vi "Derivative PCA Cycles (SubVI).vi"(8 "Derivative filter on?":bool=TRUE, 9 "Derivative LPF cutoff (Hz)":dbl=15.0, 10 "dt":dbl=50.0, 11 "Waveform (samples) in":dbl[](array[numeric])) -> (0 "AIx Related":T1={"Type (4th D ZC)"=enum."Type B", "AIx (%) (4th D ZC) "=9.808766983260572, "AP (mmHg)  (4th DZC)"=3.579441860465124}, 1 "Waveform Graph":dynamicdata(graph), 3 "Fid. Points (SDW)":T2)   [LabVIEW 2017]
uses:
  <vilib>/Analysis/NI_AAL_SigProc.lvlib
panel:
  out "SDW ZC2":dbl
  out "FoDW (Peaks)":dbl[](array[numeric])
  out "FDW (Peaks)":dbl[](array[numeric])=[27.628093409204006, 83.82448575360515, 357.5002701435206, 373.0498792154545]
  out "SDW (Peaks)":dbl[](array[numeric])
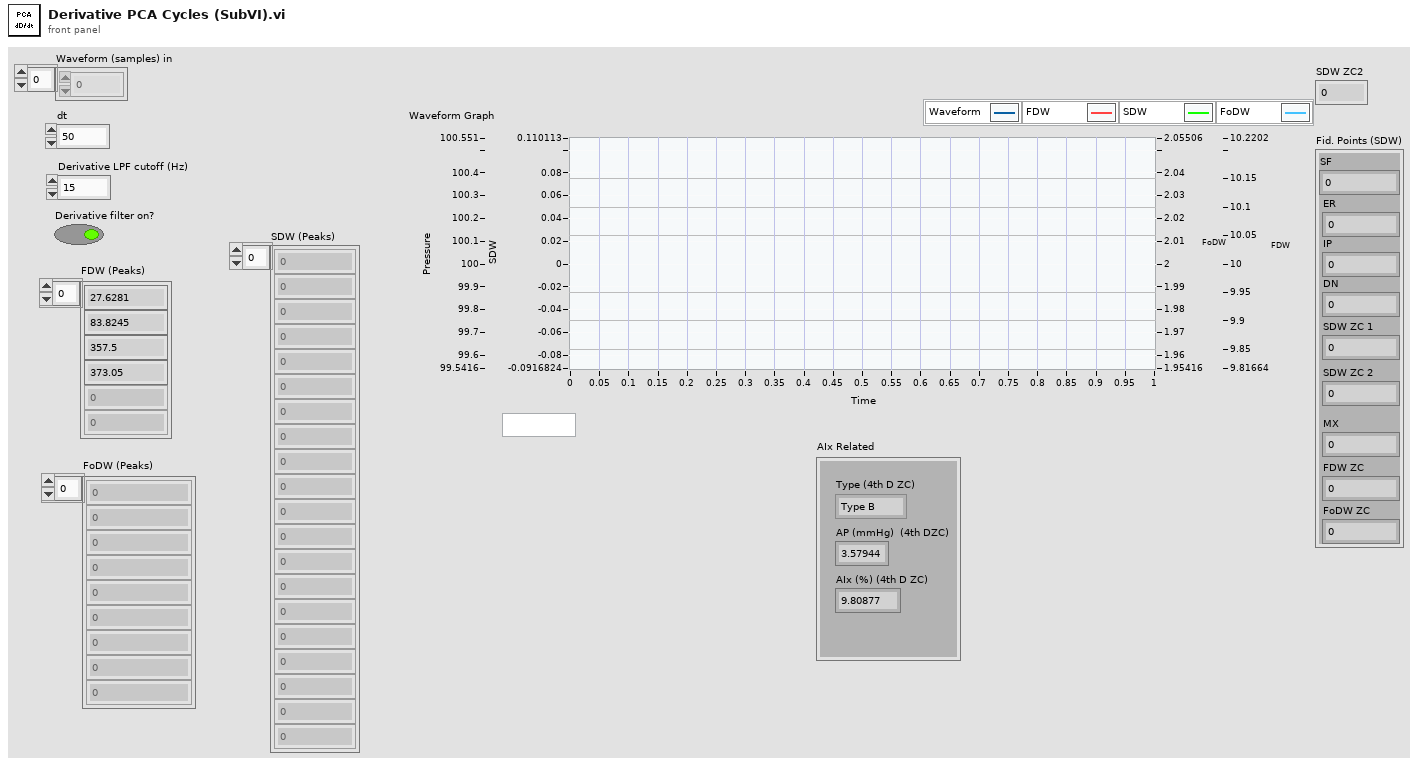
[diagram p1: front panel]
types:
  T1 = cluster{"Type (4th D ZC)":enum16{"Type A", "Type B", "Type C"}, "AIx (%) (4th D ZC) ":dbl, "AP (mmHg)  (4th DZC)":dbl}
  T2 = cluster{"SF":dbl, "ER":dbl, "IP":dbl, "DN":dbl, "SDW ZC 1":dbl, "MX":dbl, "FDW ZC":dbl, "FoDW ZC":dbl, "SDW ZC 2":dbl}
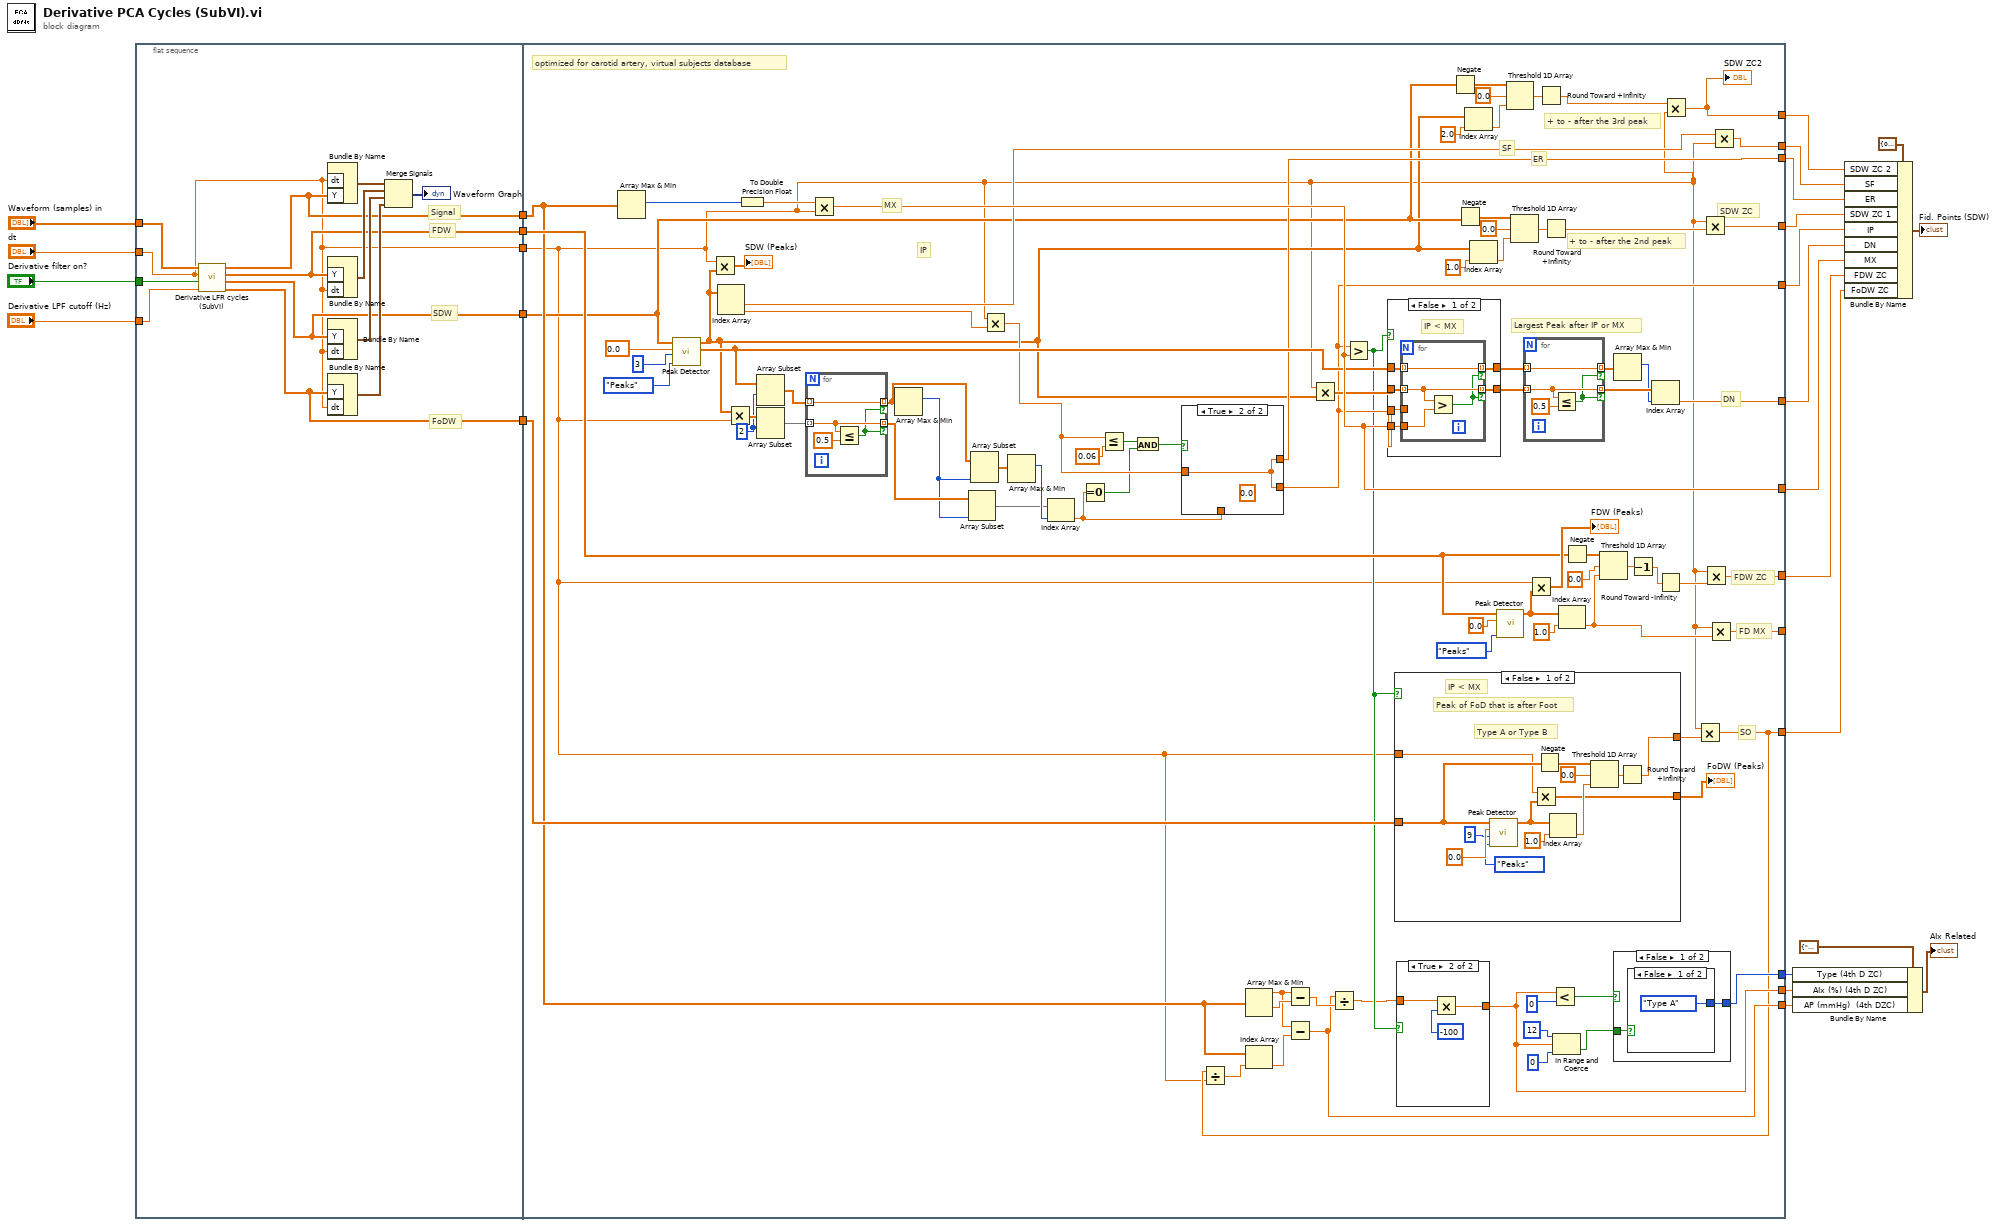
[diagram p0: block diagram]
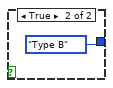
[diagram p2: hidden frame]
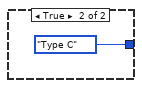
[diagram p3: hidden frame]
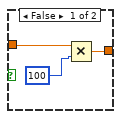
[diagram p4: hidden frame]
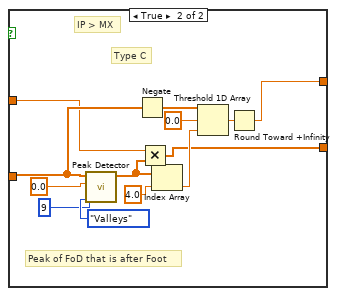
[diagram p6: hidden frame]
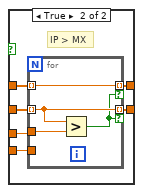
[diagram p7: hidden frame]
diagram:
  n1 = flat-sequence {
    tunnel: "Derivative LPF cutoff (Hz)" -> [w34]
    tunnel: "Derivative filter on?" -> [w36]
    tunnel: "dt" -> [w26]
    tunnel: "Waveform (samples) in" -> [w35]
    tunnel: [w30] -> w21
    tunnel: [w29] -> w20
    tunnel: [w28] -> w19
    tunnel: [w27] -> w18
    tunnel: [w26] -> w17
    tunnel: w21 -> [w65]
    tunnel: w20 -> [w101]
    tunnel: w19 -> [w43]
    tunnel: w18 -> [w98]
    tunnel: w17 -> [w40]
    tunnel: [w93] -> w16
    tunnel: [w74] -> w15
    tunnel: [w97] -> w14
    tunnel: [w96] -> w10
    tunnel: [w90] -> w12
    tunnel: [w51] -> w9
    tunnel: [w75] -> w13
    tunnel: [w95] -> w11
    tunnel: [w88] -> _
    tunnel: [w55] -> w6
    tunnel: [w54] -> w5
    tunnel: [w53] -> w4
    tunnel: [w39] -> w1
    frame #0 {
      # "FoDW"
      # "SDW"
      # "FDW"
      # "Signal"
      n2 = call "Derivative LFR cycles (SubVI).vi"("Derivative LPF cutoff (Hz)"=w34, "Derivative filter on?"=w36, "dt"=w26, "Waveform (samples) in"=w35) -> ("Fourth derivative (samples)"=w27:dbl[], "Second derivative (samples)"=w28:dbl[], "First derivative (samples)"=w29:dbl[], "Waveform (samples) out"=w30:dbl[])  [unwired: 4 in]
      n3 = Bundle By Name("dt"=w26, "Y"=w30) -> (w37:waveform(dbl))  [unwired: 1 in]
      n4 = Bundle By Name("Y"=w29, "dt"=w26) -> (w33:waveform(dbl))  [unwired: 1 in]
      n5 = Bundle By Name("Y"=w28, "dt"=w26) -> (w32:waveform(dbl))  [unwired: 1 in]
      n6 = Bundle By Name("Y"=w27, "dt"=w26) -> (w31:waveform(dbl))  [unwired: 1 in]
      n7 = Merge Signals(w37, w33, w32, w31) -> (→"Waveform Graph":dynamicdata)
    }
    frame #1 {
      w84 = 2 ("index")
      # "+ to - after the 2nd peak"
      # "+ to - after the 3rd peak"
      # "optimized for carotid artery, virtual subjects database"
      # "FD MX"
      # "ER"
      # "SF"
      # "SO"
      # "FDW ZC"
      # "SDW ZC"
      # "Largest Peak after IP or MX"
      # "MX"
      # "IP"
      # "DN"
      n8 = Array Max & Min(array=w65) -> (max index (indices)=w50:i32)  [unwired: 3 out]
      n9 = call <vilib>:"Peak Detector.vi"("peaks/valleys"=enum32{"Peaks", "Valleys"}."Peaks", "width"=3, "threshold"=0.0, "X"=w43) -> ("Amplitudes"=w85:dbl[], "Locations"=w42:dbl[])  [unwired: 3 in, 3 out]
      n10 = Multiply(x=w40, y=w42) -> (x*y=→"SDW (Peaks)":dbl[])
      n11 = Index Array(array=w42) -> (element #1=w94:dbl, element #2=w73:dbl)  [unwired: 2 in]
      n12 = Multiply(x=w42, y=w40) -> (x*y=w86:dbl[])
      n13 = To Double Precision Float(number=w50) -> (double precision float=w49:dbl)
      n14 = Array Subset(array=w85, index=w84) -> (w83:dbl[])  [unwired: 1 in]
      n15 = Array Subset(array=w86, index=w84) -> (w87:dbl[])  [unwired: 1 in]
      n16 = for {
        tunnel: w83 -> [w143] mode=indexing
        tunnel: w87 -> [w142] mode=indexing
        tunnel: [w142] -> w82 mode=indexing if=w140
        tunnel: [w143] -> w80 mode=indexing if=w140
        n17 = Less Or Equal?(x=w142, y=0.5) -> (x <= y?=w140:bool)
      }
      n18 = Multiply(x=w49, y=w40) -> (x*y=w95:dbl)
      n19 = Array Max & Min(array=w80) -> (max index (indices)=w77:i32)  [unwired: 3 out]
      n20 = Array Subset(array=w82, length=w77) -> (w78:dbl[])  [unwired: 1 in]
      n21 = Array Subset(array=w80, length=w77) -> (w79:dbl[])  [unwired: 1 in]
      n22 = Multiply(x=w40, y=w73) -> (x*y=w71:dbl)
      n23 = Array Max & Min(array=w79) -> (max index (indices)=w81:i32)  [unwired: 3 out]
      n24 = Index Array(array=w78, index=w81) -> (element=w76:dbl)
      n25 = Equal To 0?(x=w76) -> (x = 0?=w69:bool)
      n26 = Less Or Equal?(x=w71, y=0.06) -> (x <= y?=w70:bool)
      n27 = And(x=w70, y=w69) -> (x .and. y?=w68:bool)
      n28 = case shown="True" w68 {
        tunnel: w71 -> [w137 w139]
        tunnel: w76 -> [w138 _]
        tunnel: [w138 w139] -> w75
        tunnel: [w137 w139] -> w74
        frame False {
        }
        frame True {
          (unwired) 0.0 ("y")
        }
      }
      n29 = Array Max & Min(array=w65) -> (max value=w63:dbl, min value=w66:dbl)  [unwired: 2 out]
      n30 = Subtract(x=w63, y=w66) -> (x-y=w62:dbl)
      n31 = Multiply(x=w40, y=w42) -> (x*y=w92:dbl[])
      n32 = Greater?(x=w75, y=w95) -> (0:w67:bool)
      n33 = case shown="False" w67 {
        tunnel: w92 -> [w179 w189]
        tunnel: [w178 w187] -> w120
        tunnel: w75 -> [w177 w188]
        tunnel: w95 -> [w176 w186]
        tunnel: w85 -> [w175 w185]
        tunnel: [w174 w184] -> w119
        frame False {
          # "IP < MX"
          n34 = for {
            tunnel: w179 -> [w183] mode=indexing
            tunnel: w177 -> [_]
            tunnel: [w183] -> w178 mode=indexing if=w180
            tunnel: w176 -> [w182]
            tunnel: w175 -> [w181] mode=indexing
            tunnel: [w181] -> w174 mode=indexing if=w180
            n35 = Greater?(x=w183, y=w182) -> (0:w180:bool)
          }
        }
        frame True {
          # "IP > MX"
          n36 = for {
            tunnel: w189 -> [w192] mode=indexing
            tunnel: w188 -> [w193]
            tunnel: [w192] -> w187 mode=indexing if=w190
            tunnel: w186 -> [_]
            tunnel: w185 -> [w191] mode=indexing
            tunnel: [w191] -> w184 mode=indexing if=w190
            n37 = Greater?(x=w192, y=w193) -> (0:w190:bool)
          }
        }
      }
      n38 = case shown="False" w67 {
        tunnel: [w150 w165] -> w99
        tunnel: [w148 w161] -> w100
        tunnel: w98 -> [w146 w159]
        tunnel: w40 -> [w144 w157]
        frame False {
          # "IP < MX"
          # "Type A or Type B"
          # "Peak of FoD that is after Foot"
          n39 = call <vilib>:"Peak Detector.vi"("peaks/valleys"=enum32{"Peaks", "Valleys"}."Peaks", "width"=9, "threshold"=0.0, "X"=w146) -> ("Locations"=w149:dbl[])  [unwired: 3 in, 4 out]
          n40 = Multiply(x=w144, y=w149) -> (x*y=w148:dbl[])
          n41 = Negate(x=w146) -> (-x=w145:dbl[])
          n42 = Index Array(array=w149, index=1.0 ("threshold")) -> (element=w154:dbl)
          n43 = Threshold 1D Array(1:w154, 2:0.0 ("threshold y"), 3:w145) -> (0:w156:dbl)
          n44 = Round Toward +Infinity(x=w156) -> (ceil(x): smallest int >= x=w150:dbl)
        }
        frame True {
          # "IP > MX"
          # "Type C"
          # "Peak of FoD that is after Foot"
          n45 = call <vilib>:"Peak Detector.vi"("peaks/valleys"=enum32{"Peaks", "Valleys"}."Valleys", "width"=9, "threshold"=0.0, "X"=w159) -> ("Locations"=w162:dbl[])  [unwired: 3 in, 4 out]
          n46 = Negate(x=w159) -> (-x=w158:dbl[])
          n47 = Multiply(x=w157, y=w162) -> (x*y=w161:dbl[])
          n48 = Index Array(array=w162, index=4.0 ("threshold")) -> (element=w167:dbl)
          n49 = Threshold 1D Array(1:w167, 2:0.0 ("threshold y"), 3:w158) -> (0:w169:dbl)
          n50 = Round Toward +Infinity(x=w169) -> (ceil(x): smallest int >= x=w165:dbl)
        }
      }
      "FoDW (Peaks)" <- w100
      n51 = Negate(x=w43) -> (-x=w44:dbl[])
      n52 = Negate(x=w43) -> (-x=w112:dbl[])
      n53 = Index Array(array=w42, index=2.0 ("threshold")) -> (element=w48:dbl)
      n54 = Index Array(array=w42, index=1.0 ("threshold")) -> (element=w117:dbl)
      n55 = call <vilib>:"Peak Detector.vi"("peaks/valleys"=enum32{"Peaks", "Valleys"}."Peaks", "threshold"=0.0, "X"=w101) -> ("Locations"=w109:dbl[])  [unwired: 4 in, 4 out]
      n56 = Threshold 1D Array(1:w48, 2:0.0 ("threshold y"), 3:w44) -> (0:w47:dbl)
      n57 = Threshold 1D Array(1:w117, 2:0.0 ("threshold y"), 3:w112) -> (0:w116:dbl)
      n58 = for {
        tunnel: w119 -> [w173] mode=indexing
        tunnel: w120 -> [w172] mode=indexing
        tunnel: [w172] -> w121 mode=indexing if=w170
        tunnel: [w173] -> w91 mode=indexing if=w170
        n59 = Less Or Equal?(x=w172, y=0.5) -> (x <= y?=w170:bool)
      }
      n60 = Multiply(x=w40, y=w109) -> (x*y=→"FDW (Peaks)":dbl[])
      n61 = Round Toward +Infinity(x=w47) -> (ceil(x): smallest int >= x=w41:dbl)
      n62 = Round Toward +Infinity(x=w116) -> (ceil(x): smallest int >= x=w115:dbl)
      n63 = Index Array(array=w109, index=1.0 ("threshold")) -> (element=w89:dbl)
      n64 = Negate(x=w101) -> (-x=w103:dbl[])
      n65 = Threshold 1D Array(1:w89, 2:0.0 ("threshold y"), 3:w103) -> (0:w111:dbl)
      n66 = Array Max & Min(array=w91) -> (max index (indices)=w118:i32)  [unwired: 3 out]
      n67 = Decrement(x=w111) -> (x-1=w110:dbl)
      n68 = Index Array(array=w121, index=w118) -> (element=w90:dbl)
      n69 = Round Toward -Infinity(1:w110) -> (0:w102:dbl)
      n70 = Multiply(x=w41, y=w40) -> (x*y=w39:dbl)
      "SDW ZC2" <- w39
      n71 = Multiply(x=w40, y=w99) -> (x*y=w51:dbl)
      n72 = Divide(x=w51, y=w40) -> (x/y=w52:dbl)
      n73 = Index Array(array=w65, index=w52) -> (element=w64:dbl)
      n74 = Subtract(x=w63, y=w64) -> (x-y=w54:dbl)
      n75 = Divide(x=w54, y=w62) -> (x/y=w61:dbl)
      n76 = case shown="True" w67 {
        tunnel: w61 -> [w132 w136]
        tunnel: [w131 w135] -> w53
        frame False {
          n77 = Multiply(x=w132, y=100 ("index")) -> (x*y=w131:dbl)
        }
        frame True {
          n78 = Multiply(x=w136, y=-100 ("index")) -> (x*y=w135:dbl)
        }
      }
      n79 = Less?(x=w53, y=0 ("index")) -> (x < y?=w57:bool)
      n80 = In Range and Coerce(upper limit=12 ("index"), x=w53, lower limit=0 ("index")) -> (In Range?=w56:bool)  [unwired: 1 out]
      n81 = case shown="False" w57 {
        tunnel: w56 -> [w127 _]
        tunnel: [w126 enum16{"Type A", "Type B", "Type C"}."Type C"] -> w55
        frame False {
          n82 = case shown="False" w127 {
            tunnel: [enum16{"Type A", "Type B", "Type C"}."Type A" enum16{"Type A", "Type B", "Type C"}."Type B"] -> w126
            frame False {
            }
            frame True {
            }
          }
        }
        frame True {
        }
      }
      n83 = Multiply(x=w40, y=w115) -> (x*y=w97:dbl)
      n84 = Multiply(x=w40, y=w102) -> (x*y=w96:dbl)
      n85 = Multiply(x=w40, y=w89) -> (x*y=w88:dbl)
      n86 = Multiply(x=w94, y=w40) -> (x*y=w93:dbl)
    }
  }
  n87 = Bundle By Name(cluster=T1 {"Type (4th D ZC)"=enum."Type B", "AIx (%) (4th D ZC) "=11.414991114164115, "AP (mmHg)  (4th DZC)"=2.9705360824742115} ("AIx Related"), "Type (4th D ZC)"=w6, "AIx (%) (4th D ZC)"=w4, "AP (mmHg)  (4th DZC)"=w5) -> (→"AIx Related":T1)
  n88 = Bundle By Name(cluster=T2 {"SF"=0.010942260374358782, "ER"=0.06421891274775417, "IP"=0.18732576950267, "DN"=0.31391970911344796, "SDW ZC 1"=0.07, "MX"=0.116, "FDW ZC"=0.114, "FoDW ZC"=0.17200000000000001, "SDW ZC 2"=0.07} ("Fid. Points (SDW)"), "SDW ZC 2"=w1, "SF"=w16, "ER"=w15, "SDW ZC 1"=w14, "IP"=w13, "DN"=w12, "MX"=w11, "FDW ZC"=w10, "FoDW ZC"=w9) -> (→"Fid. Points (SDW)":T2)
